vi "Init.vi"(8 "error in (no error)":errorcluster, 11 "Flanger in":refnum<class "Flanger.lvclass">) -> (0 "error out":errorcluster, 3 "Flanger out":refnum<class "Flanger.lvclass">)   [LabVIEW 2019, in "Flanger.lvlib" / "Flanger.lvclass"]
uses:
  Flanger.lvclass
  Plugin Interfaces/Effect Interface/Effect Interface.lvlibp/Plugin Interfaces/Effect Interface/Effect Interface Class/Effect Interface.lvclass
  Plugin Interfaces/Effect Interface/Effect Interface.lvlibp/Libraries/Audio Processing/Value Properties.ctl
  Plugin Interfaces/Effect Interface/Effect Interface.lvlibp/Libraries/Audio Processing/Audio Processing.lvlib
  Plugin Interfaces/Effect Interface/Effect Interface.lvlibp/Libraries/Audio Processing/Value Cluster.ctl
  C:/github/dataflowg/dataflow-dj/src/Plugin Interfaces/Effect Interface/Effect Interface.lvlibp/Plugin Interfaces/Effect Interface/Effect Interface Class/Effect Interface.lvclass
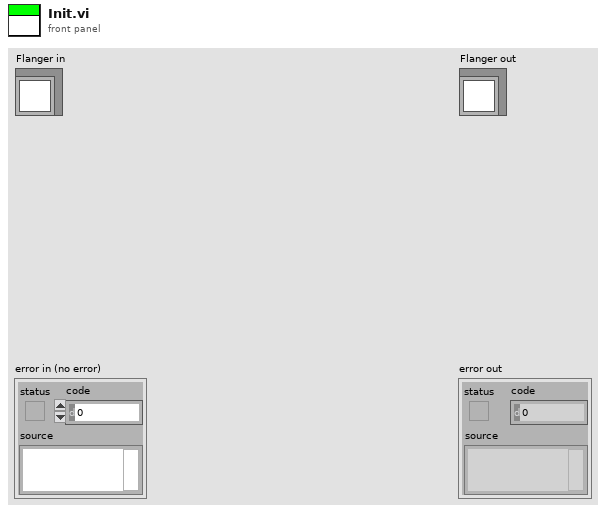
[diagram p1: front panel]
types:
  T1 = typedef "Effect Interface.lvlibp/Audio Processing.lvlib/Value Cluster.ctl" = cluster{"Value":dbl, "Properties":T2}
  T2 = typedef "Effect Interface.lvlibp/Audio Processing.lvlib/Value Properties.ctl" = cluster{"Lower":dbl, "Upper":dbl, "Default":dbl, "Increment":dbl}
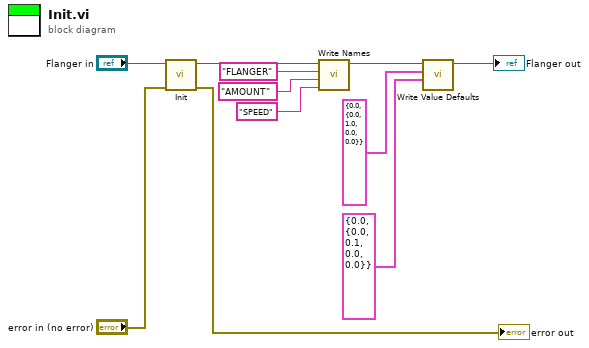
[diagram p0: block diagram]
diagram:
  n1 = call-parent "Init.vi"("error in (no error)"="error in (no error)", "Effect Interface in"="Flanger in") -> ("error out"=→"error out":errorcluster, "Effect Interface out"=w4:refnum<class "Flanger.lvclass">)  [unwired: 8 in]
  n2 = call "Write Names.vi"("Value2 Name"="SPEED" ("Value1 Name"), "Value1 Name"="AMOUNT", "Effect Name"="FLANGER", "Effect Interface in"=w4) -> ("Effect Interface out"=w8:refnum<class "Flanger.lvclass">)  [unwired: 7 in]
  n3 = call "Write Value Defaults.vi"("Value2"=T1 {"Value"=0.0, "Properties"={"Lower"=0.0, "Upper"=0.1, "Default"=0.0, "Increment"=0.0}} ("Value1"), "Value1"=T1 {"Value"=0.0, "Properties"={"Lower"=0.0, "Upper"=1.0, "Default"=0.0, "Increment"=0.0}}, "Effect Interface in"=w8) -> ("Effect Interface out"=→"Flanger out":refnum<class "Flanger.lvclass">)  [unwired: 8 in]
